vi "get reignition voltage.vi"() -> ()   [LabVIEW 2018]
uses:
  <vilib>/DAQmx/write.llb/DAQmx Write (Analog DBL 1Chan 1Samp).vi
  a8074ea1-1c0a-4296-9646-7d5559e3d868.vi
  b15d0405-1705-47a4-a36f-a0cd54eda9bd.vi
  37882e86-5f32-4f0b-bb7e-73c8138da298.vi
  <vilib>/DAQmx/read.llb/DAQmx Read (Analog DBL 1Chan 1Samp).vi
  <vilib>/DAQmx/create/channels.llb/DAQmx Create Channel (AO-Voltage-Basic).vi
  <vilib>/DAQmx/create/channels.llb/DAQmx Create Channel (AI-Voltage-Basic).vi
  <vilib>/DAQmx/miscellaneous.llb/DAQmx Fill In Error Info.vi
panel:
  out "Waveform Chart":dbl(graph)
  out "current rf voltage in":dbl
  out "Min Reignition Voltage":dbl
  in  "Reigniter":tag="Dev1/ao1"
  out "stable rf gen voltage":dbl
  out "polarimeter threshold":dbl
  in  "polarimeter":tag="Dev1/ai1"
  in  "RF Generator":tag="Dev1/ao0"
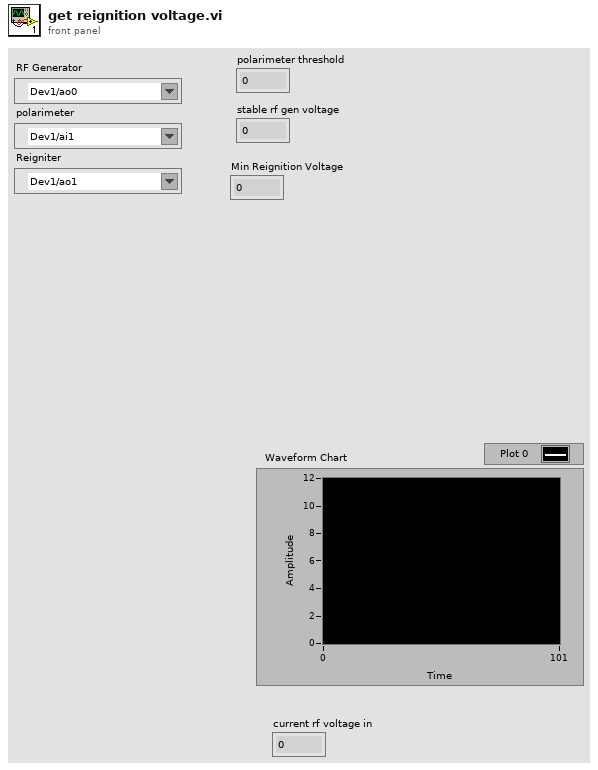
[diagram p1: front panel]
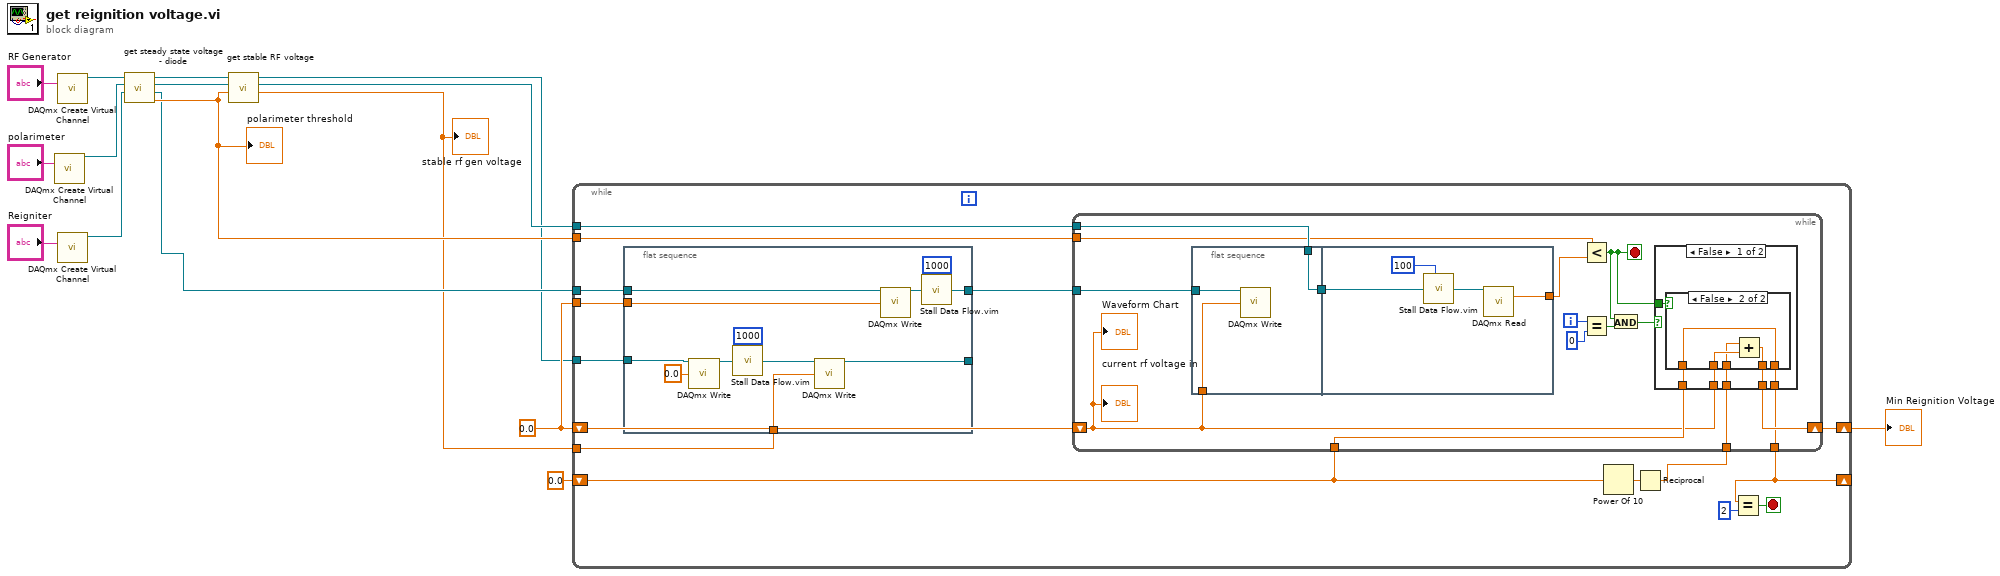
[diagram p0: block diagram]
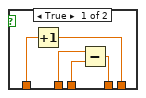
[diagram p2: hidden frame]
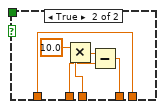
[diagram p3: hidden frame]
diagram:
  w4 = 0.0
  n1 = call-poly <vilib>:"DAQmx Create Virtual Channel.vi"("physical channels"="polarimeter") -> ("task out"=w12:refnum<k21>)  [unwired: 13 in, 1 out]
  n2 = call-poly <vilib>:"DAQmx Create Virtual Channel.vi"("physical channels"="RF Generator") -> ("task out"=w11:refnum<k21>)  [unwired: 13 in, 1 out]
  n3 = call-poly <vilib>:"DAQmx Create Virtual Channel.vi"("physical channels"="Reigniter") -> ("task out"=w13:refnum<k21>)  [unwired: 13 in, 1 out]
  n4 = call "get steady state voltage - diode.vi"("Reignition Task In"=w13, "Diode Task In"=w12, "RF Generator Task In"=w11) -> ("Output"=w6:dbl, "reignition task out"=w5:refnum<k21>, "diode task out"=w10:refnum<k21>, "rf generator task out"=w9:refnum<k21>)  [unwired: 5 in]
  "polarimeter threshold" <- w6
  n5 = call "get stable RF voltage.vi"("diode steady state voltage"=w6, "polarimeter task in"=w10, "rf gen task in"=w9) -> ("stable voltage"=w1:dbl, "polarimeter task out"=w7:refnum<k21>, "rf gen task out"=w2:refnum<k21>)  [unwired: 6 in]
  "stable rf gen voltage" <- w1
  n6 = while {
    tunnel: w7 -> [w22]
    shift-right: [w26] -> w8
    shift-left: w4 -> [w19]
    tunnel: w5 -> [w30]
    tunnel: w4 -> [w29]
    shift-right: [w23] -> _
    shift-left: 0.0 -> [w25]
    tunnel: w6 -> [w20]
    tunnel: w2 -> [w18]
    tunnel: w1 -> [w17]
    stop <- w27 stop-if-true
    n7 = flat-sequence {
      tunnel: w30 -> [w41]
      tunnel: w29 -> [w40]
      tunnel: [w39] -> w21
      tunnel: w18 -> [w34]
      tunnel: w17 -> [w33]
      tunnel: [w32] -> _
      frame #0 {
        n8 = call-poly <vilib>:"DAQmx Write.vi"("task/channels in"=w34, "data"=0.0) -> ("task out"=w37:refnum<k21>)  [unwired: 11 in, 2 out]
        n9 = call "Stall Data Flow.vim"("value in"=w37, "milliseconds to wait"=u32 1000) -> ("value out"=w38:refnum<k21>)  [unwired: 1 out]
        n10 = call-poly <vilib>:"DAQmx Write.vi"("task/channels in"=w38, "data"=w33) -> ("task out"=w32:refnum<k21>)  [unwired: 11 in, 2 out]
        n11 = call-poly <vilib>:"DAQmx Write.vi"("task/channels in"=w41, "data"=w40) -> ("task out"=w43:refnum<k21>)  [unwired: 11 in, 2 out]
        n12 = call "Stall Data Flow.vim"("value in"=w43, "milliseconds to wait"=u32 1000) -> ("value out"=w39:refnum<k21>)  [unwired: 1 out]
      }
    }
    n13 = Power Of 10(x=w25) -> (10^x=w31:dbl)
    n14 = Reciprocal(x=w31) -> (1/x=w24:dbl)
    n15 = while {
      tunnel: w22 -> [w50]
      tunnel: w21 -> [w51]
      shift-right: [w53] -> w26
      shift-left: w19 -> [w45]
      tunnel: w24 -> [w54]
      tunnel: w25 -> [w48]
      tunnel: [w52] -> w23
      tunnel: w20 -> [w44]
      i -> [w58]
      stop <- w46 stop-if-true
      n16 = flat-sequence {
        tunnel: w45 -> [w61]
        tunnel: w51 -> [w60]
        tunnel: w50 -> [w59]
        tunnel: [w59] -> w49
        tunnel: w49 -> [w64]
        tunnel: [w63] -> w47
        frame #0 {
          n17 = call-poly <vilib>:"DAQmx Write.vi"("task/channels in"=w60, "data"=w61) -> ()  [unwired: 11 in, 3 out]
        }
        frame #1 {
          n18 = call "Stall Data Flow.vim"("value in"=w64, "milliseconds to wait"=u32 100) -> ("value out"=w65:refnum<k21>)  [unwired: 1 out]
          n19 = call-poly <vilib>:"DAQmx Read.vi"("task/channels in"=w65) -> ("data"=w63:dbl)  [unwired: 12 in, 2 out]
        }
      }
      n20 = Less?(x=w44, y=w47) -> (x < y?=w46:bool)
      n21 = Equal?(x=w58, y=0) -> (x = y?=w56:bool)
      n22 = And(x=w46, y=w56) -> (x .and. y?=w55:bool)
      n23 = case shown="False" w55 {
        tunnel: w54 -> [w69 w86]
        tunnel: w45 -> [w70 w83]
        tunnel: [w71 w82] -> w53
        tunnel: w48 -> [w68 w81]
        tunnel: [w67 w81] -> w52
        tunnel: w46 -> [w66 _]
        frame False {
          n24 = case shown="False" w66 {
            tunnel: [w76 w79] -> w71
            tunnel: w70 -> [w72 w78]
            tunnel: w69 -> [w73 w77]
            tunnel: w68 -> [w75 w80]
            tunnel: [w74 w80] -> w67
            frame True {
              n25 = Increment(x=w75) -> (x+1=w74:dbl)
              n26 = Subtract(x=w72, y=w73) -> (x-y=w76:dbl)
            }
            frame False {
              n27 = Add(x=w77, y=w78) -> (x+y=w79:dbl)
            }
          }
        }
        frame True {
          n28 = Multiply(x=10.0, y=w86) -> (x*y=w84:dbl)
          n29 = Subtract(x=w84, y=w83) -> (x-y=w82:dbl)
        }
      }
      "Waveform Chart" <- w45
      "current rf voltage in" <- w45
    }
    n30 = Equal?(x=w23, y=2) -> (x = y?=w27:bool)
  }
  "Min Reignition Voltage" <- w8
